vi "DAQ.vi"() -> ()   [LabVIEW 2020]
panel:
  out "Waveform Chart":dynamicdata(graph)
  in  "stop":bool
  out "Votage (V)":dbl
  out "oscilloscope":dynamicdata(graph)
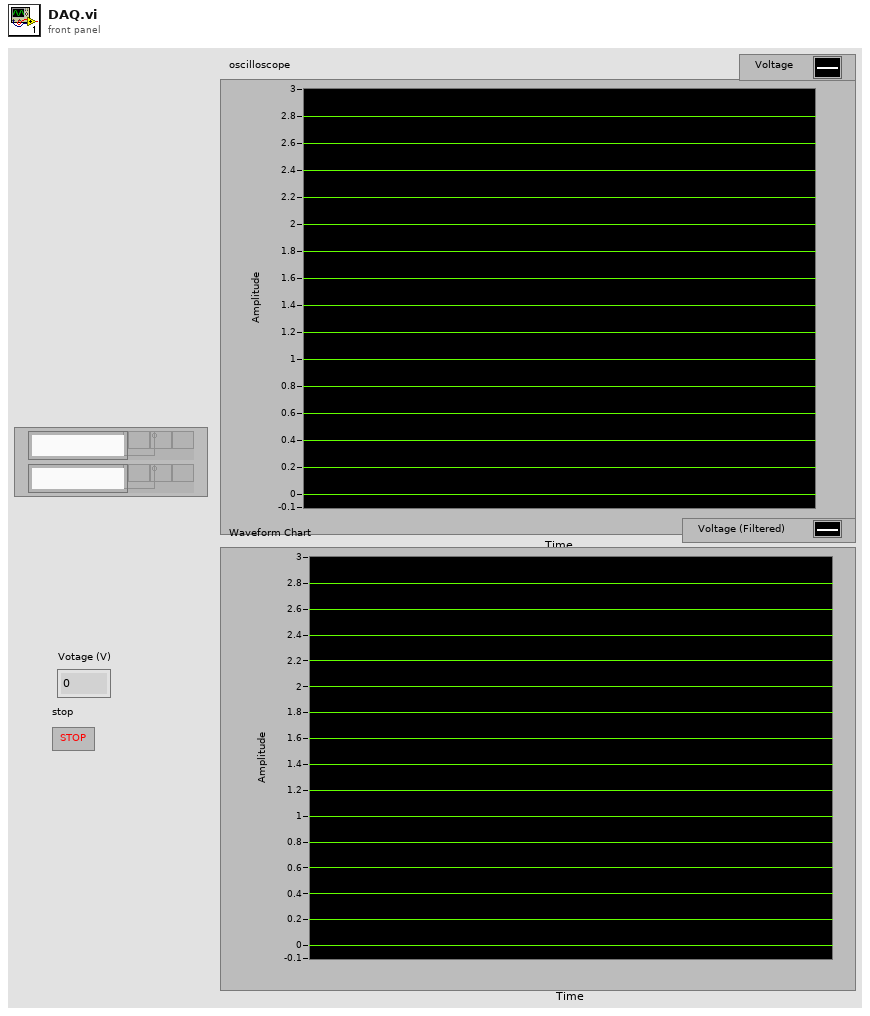
[diagram p1: front panel]
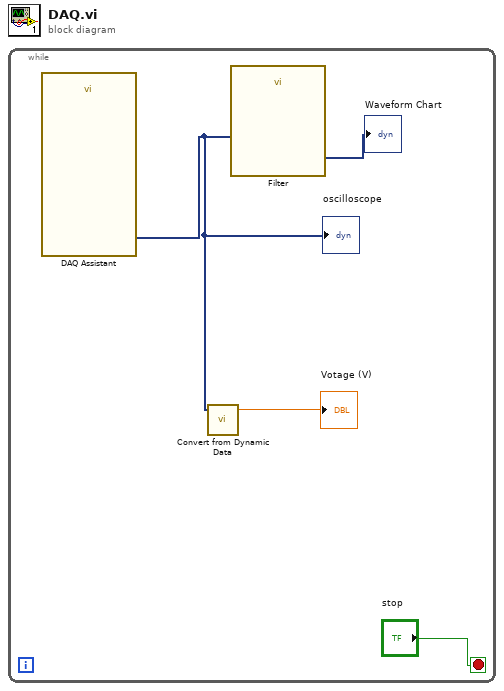
[diagram p0: block diagram]
diagram:
  n1 = while {
    stop <- "stop" stop-if-true
    n2 = call "DAQ Assistant"() -> ("data"=w2:dynamicdata)  [unwired: 16 in, 3 out]
    "oscilloscope" <- w2
    n3 = call "Convert from Dynamic Data"("Dynamic Data Type"=w2) -> ("Scalar"=→"Votage (V)":dbl)  [unwired: 3 in]
    n4 = call "Filter"("Signal"=w2) -> ("Filtered Signal"=→"Waveform Chart":dynamicdata)  [unwired: 9 in, 1 out]
  }
